vi "Begin.vi"(8 "error in":errorcluster) -> (0 "error out":errorcluster)   [LabVIEW 2017]
doc: "Called before other user functions, this VI is expected to open initial I/O refnums, load in file data, and do all program initialization. Notice that the <B>error out</B> terminal is simply used for data flow. Wiring it to other structures or subVIs ensures that this VI runs first."
uses:
  <vilib>/Rock Robotics/WPI/MotorControl/WPI_MotorControlOpen Talon.vi
  <vilib>/Rock Robotics/SystemInterfaces/DIO/FPGA_DIOPWMChannel.ctl
  <vilib>/Rock Robotics/WPI/Counter/WPI_CounterDigitalInputToDigitalSource.vi
  <vilib>/Rock Robotics/SystemInterfaces/DIO/FPGA_DIOChannel.ctl
  <vilib>/Rock Robotics/WPI/Solenoid/WPI_SolenoidOpenDouble.vi
  <vilib>/Rock Robotics/WPI/Solenoid/WPI_SolenoidChannel.ctl
  <userlib>/836-Library/Drive/Drive_Code_V2/Drive_Code_Support/SensorTypedefs/Sensor_Cluster.ctl
  <userlib>/836-Library/Drive/Drive_Code_V2/Drive_Code_Support/SensorTypedefs/Camera_Cluster.ctl
  <vilib>/Rock Robotics/WPI/RobotDrive/WPI_RobotDriveDevRef.ctl
  <vilib>/Rock Robotics/WPI/MotorControl/WPI_MotorControlDeviceRef.ctl
  <vilib>/Rock Robotics/WPI/MotorControl/WPI_MotorControlType.ctl
  <vilib>/Rock Robotics/WPI/PWM/WPI_PWMDeadband.ctl
  <userlib>/836-Library/Drive/Drive_Code_V2/Drive_Code_Support/DriveTrains/Drive_Trains.ctl
  <userlib>/836-Library/Drive/Drive_Code_V2/Drive_Code_Support/Command_Sends/Drive_Code_Command_Type.ctl
  <userlib>/836-Library/Drive/Drive_Code_V2/Drive_Code_Support/Command_Sends/Drive_Code_Command_List.ctl
  <userlib>/836-Library/Drive/Drive_Code_V2/Drive_Code_Support/PidClusters/PidInversions.ctl
  <userlib>/836-Library/Drive/Drive_Code_V2/Drive_Code_Support/PidClusters/DrivePidInputs.ctl
  <userlib>/836-Library/Drive/Drive_Code_V2/Drive_Code_Support/PidClusters/PidInputs.ctl
  <userlib>/836-Library/Drive/Drive_Code_V2/Drive_Code_Support/Command_Sends/Command_Tolerances.ctl
  <userlib>/836-Library/Drive/Drive_Code_V2/Drive_Code_Support/Command_Sends/Command_Tolerance_Info.ctl
  <userlib>/836-Library/Drive/Drive_Code_V2/Drive_Code_Support/DriveTrains/Tank/Tank_4_Motor.vi
  <userlib>/836-Library/Pneumatics/Support_Code/Pneumatics_Command.ctl
  <userlib>/836-Library/Pneumatics/Support_Code/Pneumatics_Position.ctl
  <vilib>/Rock Robotics/WPI/Solenoid/WPI_SolenoidDevRef.ctl
  <vilib>/Rock Robotics/WPI/Solenoid/WPI_SolenoidValue.ctl
  <userlib>/836-Library/Pneumatics/Support_Code/Pneumatics_Status.ctl
  <vilib>/Rock Robotics/WPI/Joystick/WPI_JoystickDeviceEnum.ctl
  <vilib>/Rock Robotics/SystemInterfaces/i2clib/i2c_bus.ctl
  <vilib>/Rock Robotics/SystemInterfaces/AI/FPGA_AIChannel.ctl
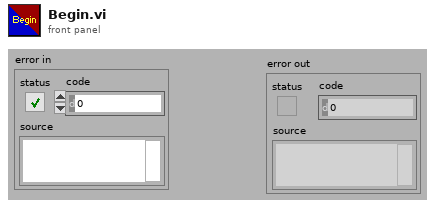
[diagram p1: front panel]
types:
  T1 = typedef "FPGA_AIChannel.ctl" = enum8{"AI 0", "AI 1", "AI 2", "AI 3", "AI MXP 0", "AI MXP 1", "AI MXP 2", "AI MXP 3", "Invalid"}
  T2 = typedef "FPGA_DIOChannel.ctl" = enum8{"DIO 0", "DIO 1", "DIO 2", "DIO 3", "DIO 4", "DIO 5", "DIO 6", "DIO 7", "DIO 8", "DIO 9", "DIO MXP 0", "DIO MXP 1", "DIO MXP 2", "DIO MXP 3", "DIO MXP 4", "DIO MXP 5", "DIO MXP 6", "DIO MXP 7", "DIO MXP 8", "DIO MXP 9", "DIO MXP 10", "DIO MXP 11", "DIO MXP 12", "DIO MXP 13", "DIO MXP 14", "DIO MXP 15", "SPI Port CS1", "SPI Port CS2", "SPI Port CS3", "SPI Port MISO", "SPI Port MOSI", "Invalid"}
  T3 = typedef "i2c_bus.ctl" = enum16{"I2C On-Board", "I2C MXP", "Invalid"}
  T4 = enum8{"ConfigMode", "AccOnly", "MagOnly", "GyroOnly", "AccMag", "AccGyro", "MagGyro", "AMG", "IMU", "Compass", "M4G", "NDOF_FMC_OFF", "NDOF"}
  T5 = typedef "WPI_JoystickDeviceEnum.ctl" = enum16{"USB 0", "USB 1", "USB 2", "USB 3", "USB 4", "USB 5"}
  T6 = typedef "WPI_SolenoidChannel.ctl" = enum8{"Solenoid 0", "Solenoid 1", "Solenoid 2", "Solenoid 3", "Solenoid 4", "Solenoid 5", "Solenoid 6", "Solenoid 7", "Invalid"}
  T7 = typedef "FPGA_DIOPWMChannel.ctl" = enum8{"PWM 0", "PWM 1", "PWM 2", "PWM 3", "PWM 4", "PWM 5", "PWM 6", "PWM 7", "PWM 8", "PWM 9", "PWM MXP 0", "PWM MXP 1", "PWM MXP 2", "PWM MXP 3", "PWM MXP 4", "PWM MXP 5", "PWM MXP 6", "PWM MXP 7", "PWM MXP 8", "PWM MXP 9", "Invalid"}
  T8 = typedef "WPI_MotorControlDeviceRef.ctl" = cluster{"DeviceStatus":errorcluster, "Type":T9, "PWM":cluster{"PWM Channel":T7, "DeadBand":T10}, "CAN":cluster{"Device Number":u8, "SetOutput VI Ref":variant, "GetOutput VI Ref":variant, "Enable VI Ref":variant, "Disable VI Ref":variant, "Data":variant}, "Invert":bool, "DIO PWM":cluster{"PWM \"Enable\" Channel":T7, "DIOChannel":T2, "PWM Rate":dbl}}
  T9 = typedef "WPI_MotorControlType.ctl" = enum16{"PWM", "CAN", "DIO PWM"}
  T10 = typedef "WPI_PWMDeadband.ctl" = cluster{"Name":string, "maxPositivePwm":i32, "minPositivePwm":i32, "centerPwm":i32, "maxNegativePwm":i32, "minNegativePwm":i32, "angularRange":u16}
  T11 = typedef "Drive_Code_Bundle.ctl" = cluster{"Sensor Data":T12, "RobotDriveDevRef":T14, "Drive Train":T15, "Valid Commands":bool[], "Drive Comand Notifier":refnum<notifier>, "Command Finished?":refnum<k4>, "Command Canceled":refnum<k4>, "PID Inversions":T16, "PID Inputs Notifier":refnum<notifier>, "Cmd Tol Notifier":refnum<notifier>}
  T12 = typedef "Sensor_Cluster.ctl" = cluster{"Gyro Data":cluster{"Gyro RT FIFO":refnum<k33>, "Gyro Current":dbl, "Gyro Hold":dbl}, "Encoder Data":cluster{"Encoder RT FIFO":refnum<k33>, "Encoder Current":dbl, "Encoder Hold":dbl}, "Camera Data":cluster{"Camera RT FIFO":refnum<k33>, "Camera Current":T13}}
  T13 = typedef "Camera_Cluster.ctl" = cluster{" Angle":dbl, "Valid":bool}
  T14 = typedef "WPI_RobotDriveDevRef.ctl" = cluster{"DevStatus":errorcluster, "Motors[]":T8[], "Square Inputs":bool, "Max Output":dbl}
  T15 = typedef "Drive_Trains.ctl" = enum16{"Tank Drive 2 Motor", "Tank Drive 4 Motor", "Tank Drive 6 Motor", "Mecanum Drive", "Kiwi Drive", "Invalid"}
  T16 = typedef "PidInversions.ctl" = cluster{"Distance PID Inverted?":bool, "Yaw PID Inverted?":bool}
  T17 = typedef "WPI_DigitalInputDevRef.ctl" = cluster{"DevStatus":errorcluster, "DIO Channel":T2}
  T18 = typedef "WPI_JoystickDevRef.ctl" = cluster{"Device":T5}
  T19 = typedef "FPGA_CounterEncoderSourceConvertionLVSourceType.ctl" = cluster{"DevStatus":errorcluster, "AnalogTriggerMode?":bool, "DigitalMode":cluster{"DIO Channel":T20}, "AnalogTriggerMode":cluster{"AnalogTriggerIndex":T21, "OutputType":T22}}
  T20 = typedef "FPGA_DIODigitalSourceChannel.ctl" = enum8{"DIO 0", "DIO 1", "DIO 2", "DIO 3", "DIO 4", "DIO 5", "DIO 6", "DIO 7", "DIO 8", "DIO 9", "DIO MXP 0", "DIO MXP 1", "DIO MXP 2", "DIO MXP 3", "DIO MXP 4", "DIO MXP 5", "DIO MXP 6", "DIO MXP 7", "DIO MXP 8", "DIO MXP 9", "DIO MXP 10", "DIO MXP 11", "DIO MXP 12", "DIO MXP 13", "DIO MXP 14", "DIO MXP 15", "Disabled"}
  T21 = typedef "FPGA_AnalogTriggerIndex.ctl" = enum8{"Trig 0", "Trig 1", "Trig 2", "Trig 3", "Trig 4", "Trig 5", "Trig 6", "Trig 7", "Invalid"}
  T22 = typedef "FPGA_AnalogTriggerOutType.ctl" = enum16{"InWindow", "TriggerState", "Rising", "Falling"}
  T23 = typedef "WPI_SolenoidDevRef.ctl" = cluster{"DevStatus":errorcluster, "Pneumatics Control Module":u8, "Forward Solenoid Channel":T6, "Reverse Solenoid Channel":T6}
  T24 = typedef "WPI_EncoderDevRef.ctl" = cluster{"DevStatus":errorcluster, "EncoderIndex":T25, "CounterIndex":T26, "DistancePerCount":dbl, "Decoding Type":T27}
  T25 = typedef "FPGA_EncoderIdx.ctl" = enum8{"Enc 0", "Enc 1", "Enc 2", "Enc 3", "Enc 4", "Enc 5", "Enc 6", "Enc 7", "Invalid"}
  T26 = typedef "FPGA_CounterCtrSystemIndex.ctl" = enum8{"Ctr 0", "Ctr 1", "Ctr 2", "Ctr 3", "Ctr 4", "Ctr 5", "Ctr 6", "Ctr 7", "Invalid"}
  T27 = typedef "WPI_EncoderType.ctl" = enum16{"1x", "2x", "4x"}
  T28 = typedef "ImuDevRef.ctl" = cluster{"I2CDevRef":T29, "Valid Cal File?":bool}
  T29 = typedef "WPI_I2CDevRef.ctl" = cluster{"DevStatus":errorcluster, "Device Address":u8, "Handle":i32, "I2C Bus":T3}
  T30 = typedef "Pneumatics_Notifier.ctl" = cluster{"Command":refnum<notifier>, "Status":refnum<queue>}
  T31 = typedef "Pneumatic_Sensor_Loop.ctl" = cluster{"Status Queue":refnum<queue>, "Status Loop":refnum<k33>, "Relay Value":T32}
  T32 = typedef "WPI_SolenoidValue.ctl" = enum16{"Off", "On", "Forward", "Reverse"}
  T33 = typedef "Solenoid_Control_Loop.ctl" = cluster{"Control Notifier":refnum<notifier>, "Initial Position":T34, "SolenoidDevRef":T23, "Status Loop":refnum<k33>}
  T34 = typedef "Pneumatics_Position.ctl" = enum16{"Forward", "Reverse"}
  T35 = typedef "WPI_AnalogChannelDevRef.ctl" = cluster{"DevStatus":errorcluster, "Analog Channel":T1}
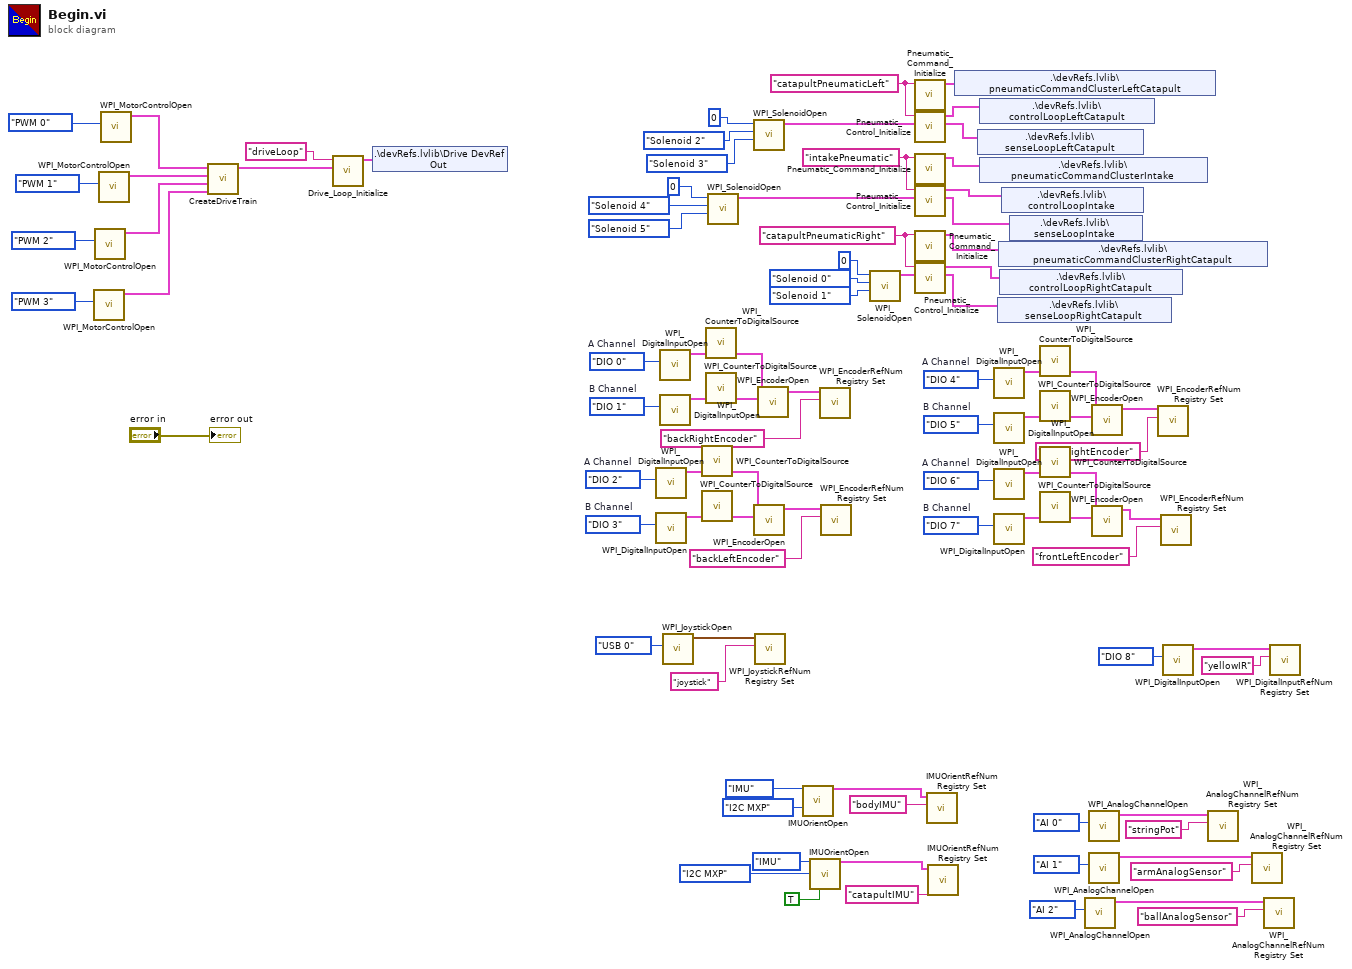
[diagram p0: block diagram]
diagram:
  w32 = FPGA_DIOChannel."DIO 7"  # B Channel
  w33 = FPGA_DIOChannel."DIO 6"  # A Channel
  w43 = FPGA_DIOChannel."DIO 5"  # B Channel
  w42 = FPGA_DIOChannel."DIO 4"  # A Channel
  w44 = FPGA_DIOChannel."DIO 3"  # B Channel
  w45 = FPGA_DIOChannel."DIO 2"  # A Channel
  w73 = "catapultPneumaticRight" ("name (unnamed)")
  w72 = "catapultPneumaticLeft" ("name (unnamed)")
  w74 = "intakePneumatic" ("name (unnamed)")
  w80 = FPGA_DIOChannel."DIO 1"  # B Channel
  w79 = FPGA_DIOChannel."DIO 0"  # A Channel
  n1 = call-poly <vilib>:"WPI_MotorControlOpen.vi"("PWM Channel"=FPGA_DIOPWMChannel."PWM 3") -> ("MotorControlDeviceRef"=w88:T8)  [unwired: 9 in, 1 out]
  n2 = call-poly <vilib>:"WPI_MotorControlOpen.vi"("PWM Channel"=FPGA_DIOPWMChannel."PWM 2") -> ("MotorControlDeviceRef"=w89:T8)  [unwired: 9 in, 1 out]
  n3 = call-poly <vilib>:"WPI_MotorControlOpen.vi"("PWM Channel"=FPGA_DIOPWMChannel."PWM 1") -> ("MotorControlDeviceRef"=w90:T8)  [unwired: 9 in, 1 out]
  n4 = call-poly <vilib>:"WPI_MotorControlOpen.vi"("PWM Channel"=FPGA_DIOPWMChannel."PWM 0") -> ("MotorControlDeviceRef"=w91:T8)  [unwired: 9 in, 1 out]
  n5 = call-poly <userlib>:"CreateDriveTrain.vi"("Front Right Motor"=w88, "Front Left Motor"=w89, "Rear Right Motor"=w90, "Rear Left Motor"=w91) -> ("DriveClusterOut"=w83:T11)  [unwired: 7 in]
  n6 = call <userlib>:"Drive_Loop_Initialize.vi"("Drive Train Ref"=w83, "Name"="driveLoop") -> ("Drive DevRef Out"=w81:T11)  [unwired: 9 in]
  n7 = shared-variable ".\\devRefs.lvlib\\Drive DevRef Out"(w81) -> ()  [unwired: 1 in, 1 out]
  n8 = call <vilib>:"WPI_DigitalInputOpen.vi"("DIO Channel"=w45) -> ("DigitalInputDevRef"=w48:T17)  [unwired: 1 in, 9 out]
  n9 = call <vilib>:"WPI_DigitalInputOpen.vi"("DIO Channel"=w44) -> ("DigitalInputDevRef"=w47:T17)  [unwired: 1 in, 9 out]
  n10 = call <vilib>:"WPI_DigitalInputOpen.vi"("DIO Channel"=w79) -> ("DigitalInputDevRef"=w76:T17)  [unwired: 1 in, 9 out]
  n11 = call <vilib>:"WPI_DigitalInputOpen.vi"("DIO Channel"=w80) -> ("DigitalInputDevRef"=w77:T17)  [unwired: 1 in, 9 out]
  n12 = call <vilib>:"WPI_JoystickOpen.vi"("JoystickDevice"=WPI_JoystickDeviceEnum."USB 0") -> ("JoystickDevRef"=w22:T18)  [unwired: 10 in]
  n13 = call-poly <vilib>:"WPI_CounterToDigitalSource.vi"("DigitalInputDevRef"=w48) -> ("Digital Source"=w49:T19)  [unwired: 6 out]
  n14 = call-poly <vilib>:"WPI_CounterToDigitalSource.vi"("DigitalInputDevRef"=w47) -> ("Digital Source"=w46:T19)  [unwired: 6 out]
  n15 = call-poly <vilib>:"WPI_CounterToDigitalSource.vi"("DigitalInputDevRef"=w76) -> ("Digital Source"=w75:T19)  [unwired: 6 out]
  n16 = call-poly <vilib>:"WPI_CounterToDigitalSource.vi"("DigitalInputDevRef"=w77) -> ("Digital Source"=w78:T19)  [unwired: 6 out]
  n17 = call-poly <vilib>:"WPI_SolenoidOpen.vi"("Reverse Solenoid Channel"=WPI_SolenoidChannel."Solenoid 5", "Forward Solenoid Channel"=WPI_SolenoidChannel."Solenoid 4", "Pneumatics Control Module (0)"=u8 0) -> ("SolenoidDevRef"=w70:T23)  [unwired: 7 in, 1 out]
  n18 = call-poly <vilib>:"WPI_SolenoidOpen.vi"("Reverse Solenoid Channel"=WPI_SolenoidChannel."Solenoid 3", "Forward Solenoid Channel"=WPI_SolenoidChannel."Solenoid 2", "Pneumatics Control Module (0)"=u8 0) -> ("SolenoidDevRef"=w71:T23)  [unwired: 7 in, 1 out]
  n19 = call <vilib>:"WPI_EncoderOpen.vi"("BSource"=w46, "ASource"=w49) -> ("EncoderDevRef"=w30:T24)  [unwired: 6 in, 3 out]
  n20 = call <vilib>:"WPI_JoystickRefNum Registry Set.vi"("refnum name"="joystick", "JoystickDevRef"=w22) -> ()  [unwired: 8 in, 2 out]
  n21 = call <vilib>:"WPI_EncoderOpen.vi"("BSource"=w78, "ASource"=w75) -> ("EncoderDevRef"=w31:T24)  [unwired: 6 in, 3 out]
  n22 = call <userlib>:"IMUOrientOpen.vi"("Op Mode"=T4."IMU", "I2C Bus"=i2c_bus."I2C MXP") -> ("IMU Dev Ref"=w18:T28)  [unwired: 7 in, 6 out]
  n23 = call <userlib>:"IMUOrientOpen.vi"("Op Mode"=T4."IMU", "I2C Bus"=i2c_bus."I2C MXP", "Alt Adr?"=TRUE) -> ("IMU Dev Ref"=w19:T28)  [unwired: 6 in, 6 out]
  n24 = call <vilib>:"WPI_EncoderRefNum Registry Set.vi"("refnum name"="backRightEncoder", "EncoderDevRef"=w31) -> ()  [unwired: 8 in, 2 out]
  n25 = call <vilib>:"WPI_EncoderRefNum Registry Set.vi"("refnum name"="backLeftEncoder", "EncoderDevRef"=w30) -> ()  [unwired: 8 in, 2 out]
  n26 = call-poly <vilib>:"WPI_SolenoidOpen.vi"("Reverse Solenoid Channel"=WPI_SolenoidChannel."Solenoid 1", "Forward Solenoid Channel"=WPI_SolenoidChannel."Solenoid 0", "Pneumatics Control Module (0)"=u8 0) -> ("SolenoidDevRef"=w69:T23)  [unwired: 7 in, 1 out]
  n27 = call <userlib>:"Pneumatic_Command_Initialize.vi"("name (unnamed)"=w72) -> ("Pneumatic Command Cluster"=w59:T30)  [unwired: 9 in, 1 out]
  n28 = call <userlib>:"Pneumatic_Control_Initialize.vi"("SolenoidDevRef"=w71, "name (unnamed)"=w72) -> ("Sense Loop"=w57:T31, "Control Loop"=w58:T33)  [unwired: 8 in]
  n29 = call <userlib>:"Pneumatic_Command_Initialize.vi"("name (unnamed)"=w74) -> ("Pneumatic Command Cluster"=w56:T30)  [unwired: 9 in, 1 out]
  n30 = call <userlib>:"Pneumatic_Control_Initialize.vi"("SolenoidDevRef"=w70, "name (unnamed)"=w74) -> ("Sense Loop"=w54:T31, "Control Loop"=w55:T33)  [unwired: 8 in]
  n31 = call <userlib>:"Pneumatic_Command_Initialize.vi"("name (unnamed)"=w73) -> ("Pneumatic Command Cluster"=w53:T30)  [unwired: 9 in, 1 out]
  n32 = call <userlib>:"Pneumatic_Control_Initialize.vi"("SolenoidDevRef"=w69, "name (unnamed)"=w73) -> ("Sense Loop"=w51:T31, "Control Loop"=w52:T33)  [unwired: 8 in]
  n33 = call <userlib>:"IMUOrientRefNum Registry Set.vi"("refnum name"="bodyIMU", "IMUDevRef in"=w18) -> ()  [unwired: 8 in, 2 out]
  n34 = call <userlib>:"IMUOrientRefNum Registry Set.vi"("refnum name"="catapultIMU", "IMUDevRef in"=w19) -> ()  [unwired: 8 in, 2 out]
  n35 = shared-variable ".\\devRefs.lvlib\\pneumaticCommandClusterLeftCatapult"(w59) -> ()  [unwired: 1 in, 1 out]
  n36 = shared-variable ".\\devRefs.lvlib\\senseLoopLeftCatapult"(w57) -> ()  [unwired: 1 in, 1 out]
  n37 = shared-variable ".\\devRefs.lvlib\\controlLoopLeftCatapult"(w58) -> ()  [unwired: 1 in, 1 out]
  n38 = shared-variable ".\\devRefs.lvlib\\pneumaticCommandClusterIntake"(w56) -> ()  [unwired: 1 in, 1 out]
  n39 = call <vilib>:"WPI_DigitalInputOpen.vi"("DIO Channel"=w42) -> ("DigitalInputDevRef"=w39:T17)  [unwired: 1 in, 9 out]
  n40 = call <vilib>:"WPI_DigitalInputOpen.vi"("DIO Channel"=w43) -> ("DigitalInputDevRef"=w40:T17)  [unwired: 1 in, 9 out]
  n41 = call <vilib>:"WPI_DigitalInputOpen.vi"("DIO Channel"=w33) -> ("DigitalInputDevRef"=w36:T17)  [unwired: 1 in, 9 out]
  n42 = call <vilib>:"WPI_DigitalInputOpen.vi"("DIO Channel"=w32) -> ("DigitalInputDevRef"=w35:T17)  [unwired: 1 in, 9 out]
  n43 = shared-variable ".\\devRefs.lvlib\\senseLoopRightCatapult"(w51) -> ()  [unwired: 1 in, 1 out]
  n44 = shared-variable ".\\devRefs.lvlib\\pneumaticCommandClusterRightCatapult"(w53) -> ()  [unwired: 1 in, 1 out]
  n45 = shared-variable ".\\devRefs.lvlib\\controlLoopRightCatapult"(w52) -> ()  [unwired: 1 in, 1 out]
  n46 = shared-variable ".\\devRefs.lvlib\\controlLoopIntake"(w55) -> ()  [unwired: 1 in, 1 out]
  n47 = shared-variable ".\\devRefs.lvlib\\senseLoopIntake"(w54) -> ()  [unwired: 1 in, 1 out]
  n48 = call-poly <vilib>:"WPI_CounterToDigitalSource.vi"("DigitalInputDevRef"=w39) -> ("Digital Source"=w38:T19)  [unwired: 6 out]
  n49 = call-poly <vilib>:"WPI_CounterToDigitalSource.vi"("DigitalInputDevRef"=w40) -> ("Digital Source"=w41:T19)  [unwired: 6 out]
  n50 = call-poly <vilib>:"WPI_CounterToDigitalSource.vi"("DigitalInputDevRef"=w36) -> ("Digital Source"=w37:T19)  [unwired: 6 out]
  n51 = call-poly <vilib>:"WPI_CounterToDigitalSource.vi"("DigitalInputDevRef"=w35) -> ("Digital Source"=w34:T19)  [unwired: 6 out]
  n52 = call <vilib>:"WPI_AnalogChannelOpen.vi"("Analog Channel"=FPGA_AIChannel."AI 2") -> ("AIDeviceRef"=w4:T35)  [unwired: 9 in, 1 out]
  n53 = call <vilib>:"WPI_AnalogChannelOpen.vi"("Analog Channel"=FPGA_AIChannel."AI 0") -> ("AIDeviceRef"=w3:T35)  [unwired: 9 in, 1 out]
  n54 = call <vilib>:"WPI_AnalogChannelOpen.vi"("Analog Channel"=FPGA_AIChannel."AI 1") -> ("AIDeviceRef"=w9:T35)  [unwired: 9 in, 1 out]
  n55 = call <vilib>:"WPI_EncoderOpen.vi"("BSource"=w41, "ASource"=w38) -> ("EncoderDevRef"=w26:T24)  [unwired: 6 in, 3 out]
  n56 = call <vilib>:"WPI_EncoderOpen.vi"("BSource"=w34, "ASource"=w37) -> ("EncoderDevRef"=w25:T24)  [unwired: 6 in, 3 out]
  n57 = call <vilib>:"WPI_EncoderRefNum Registry Set.vi"("refnum name"="frontRightEncoder", "EncoderDevRef"=w26) -> ()  [unwired: 8 in, 2 out]
  n58 = call <vilib>:"WPI_EncoderRefNum Registry Set.vi"("refnum name"="frontLeftEncoder", "EncoderDevRef"=w25) -> ()  [unwired: 8 in, 2 out]
  n59 = call <vilib>:"WPI_DigitalInputOpen.vi"("DIO Channel"=FPGA_DIOChannel."DIO 8") -> ("DigitalInputDevRef"=w11:T17)  [unwired: 9 in, 1 out]
  n60 = call <vilib>:"WPI_AnalogChannelRefNum Registry Set.vi"("refnum name"="stringPot", "AIDeviceRef"=w3) -> ()  [unwired: 8 in, 2 out]
  n61 = call <vilib>:"WPI_AnalogChannelRefNum Registry Set.vi"("refnum name"="armAnalogSensor", "AIDeviceRef"=w9) -> ()  [unwired: 8 in, 2 out]
  n62 = call <vilib>:"WPI_AnalogChannelRefNum Registry Set.vi"("refnum name"="ballAnalogSensor", "AIDeviceRef"=w4) -> ()  [unwired: 8 in, 2 out]
  n63 = call <vilib>:"WPI_DigitalInputRefNum Registry Set.vi"("refnum name"="yellowIR", "DigitalInputDevRef"=w11) -> ()  [unwired: 8 in, 2 out]
  "error out" <- "error in"
